vi "GetChildren.vi"(8 "error in (no error)":errorcluster, 10 "Parent Tag":string, 11 "TreeControl in":refnum<vi>) -> (0 "error out":errorcluster, 2 "Children Tag":string[](array[string]), 3 "TreeControl out":refnum<vi>)   [LabVIEW 2020, in "TreeControlLib.lvlib"]
uses:
  TreeControlLib.lvlib
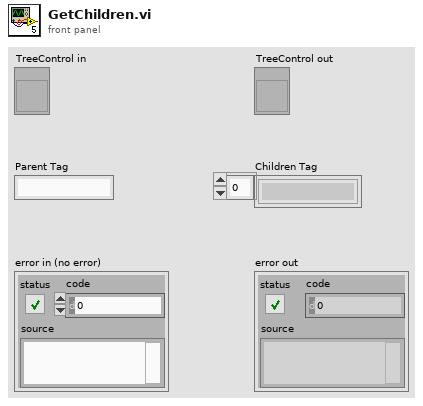
[diagram p1: front panel]
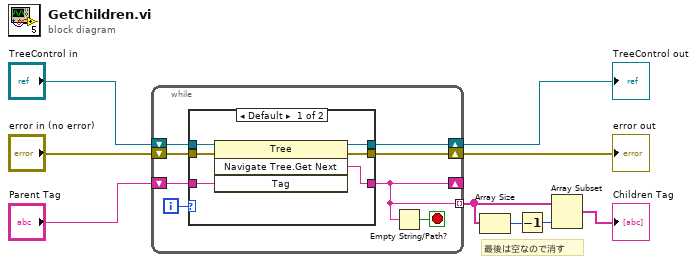
[diagram p0: block diagram]
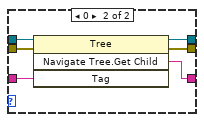
[diagram p2: hidden frame]
diagram:
  # "最後は空なので消す"
  n1 = while {
    shift-right: [w13] -> w8
    shift-left: "TreeControl in" -> [w17]
    shift-right: [w12] -> w9
    shift-left: "error in (no error)" -> [w16]
    shift-right: [w11] -> _
    shift-left: "Parent Tag" -> [w15]
    tunnel: [w11] -> w2 mode=indexing
    i -> [w14]
    stop <- w10 stop-if-true
    n2 = case shown="Default" w14 {
      tunnel: w17 -> [w23 w29]
      tunnel: [w21 w28] -> w13
      tunnel: w16 -> [w22 w27]
      tunnel: [w20 w26] -> w12
      tunnel: w15 -> [w19 w25]
      tunnel: [w18 w24] -> w11
      frame Default {
        n3 = invoke class="Tree" method="Navigate Tree.Get Next"(reference=w23, error in=w22, "Tag"=w19) -> (reference out=w21:refnum<vi>, error out=w20:errorcluster, "Navigate Tree:Get Next Item"=w18:string)  [unwired: 1 in, 1 out]
      }
      frame 0 {
        n4 = invoke class="Tree" method="Navigate Tree.Get Child"(reference=w29, error in=w27, "Tag"=w25) -> (reference out=w28:refnum<vi>, error out=w26:errorcluster, "Navigate Tree:Get Child"=w24:string)  [unwired: 1 in, 1 out]
      }
    }
    n5 = Empty String/Path?(string/path=w11) -> (empty?=w10:bool)
  }
  "error out" <- w9
  "TreeControl out" <- w8
  n6 = Array Size(array=w2) -> (size(s)=w3:i32)
  n7 = Decrement(x=w3) -> (x-1=w1:i32)
  n8 = Array Subset(array=w2, length=w1) -> (→"Children Tag":string[])  [unwired: 1 in]
